vi "Read Tree Menu Plugin Entries.vi"(4 "Error In":errorcluster, 6 "Menu Context":T1, 7 "Config Data_DB_JET in":refnum<class "Config Data_DB_ADO_Jet.lvclass">) -> (0 "Error Out":errorcluster, 2 "Tree Menu Plugin Entries":T2[](array[typedef]), 3 "Config Data_DB_JET out":refnum<class "Config Data_DB_ADO_Jet.lvclass">)   [LabVIEW 2020, in "Config Data.lvlib" / "Config Data_DB_ADO_Jet.lvclass"]
uses:
  Config Data_DB_ADO_Jet.lvclass
  C:/Users/Fred Guo/Desktop/Release 19/_libraries/Config Data/DB/Config Data_DB.lvclass
  typedefs/Tree Menu Entry.ctl
  typedefs/Menu Context Selections.ctl
  toolbox/ADO Database Drivers/ADO Database Drivers.lvlib
  Config Data_DB.lvclass
  Config Data.lvclass
  Config Data_DB_ADO.lvclass
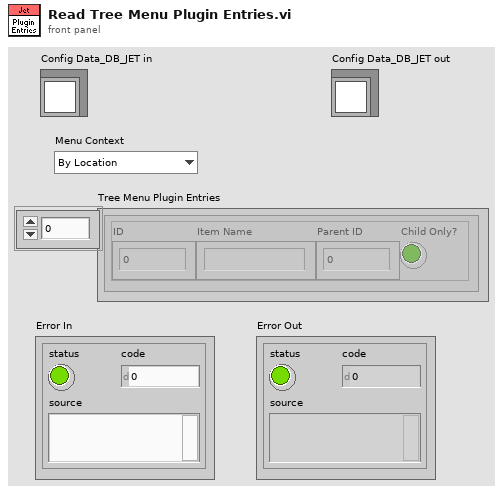
[diagram p1: front panel]
types:
  T1 = typedef "Config Data.lvlib/Config Data.lvclass/Menu Context Selections.ctl" = enum16{"By Location", "By Function"}
  T2 = typedef "Config Data.lvlib/Config Data.lvclass/Tree Menu Entry.ctl" = cluster{"ID":i32, "Item Name":string, "Parent ID":i32, "Child Only?":bool}
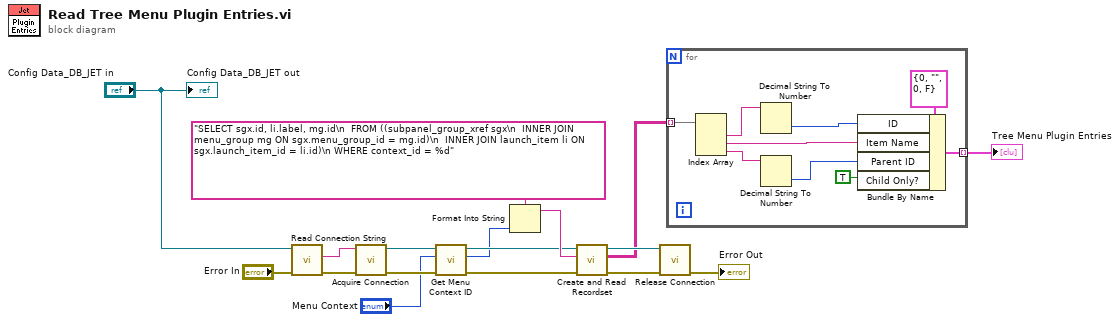
[diagram p0: block diagram]
diagram:
  n1 = call "Read Connection String.vi"("Error In"="Error In", "DB In"="Config Data_DB_JET in") -> ("Error Out"=w14:errorcluster, "Connection String"=w13:string)  [unwired: 3 in, 1 out]
  n2 = call "Acquire Connection.vi"("error in (no error)"=w14, "Connection String"=w13) -> ("error out"=w5:errorcluster, "Connection"=w6:refnum<k7>)  [unwired: 3 in, 1 out]
  n3 = call "Get Menu Context ID.vi"("error in (no error)"=w5, "Menu Context"="Menu Context", "Connection In"=w6) -> ("error out"=w4:errorcluster, "context_id"=w2:i32, "Connection Out"=w3:refnum<k7>)  [unwired: 2 in]
  n4 = Format Into String(format string="SELECT sgx.id, li.label, mg.id\n  FROM ((subpanel_group_xref sgx\n  INNER JOIN menu_group mg ON sgx.menu_group_id = mg.id)\n  INNER JOIN launch_item li ON sgx.launch_item_id = li.id)\n WHERE context_id = %d", w2) -> (resulting string=w12:string)  [unwired: 2 in, 1 out]
  n5 = call "Create and Read Recordset.vi"("error in (no error)"=w4, "Source"=w12, "Connection In"=w3) -> ("error out"=w17:errorcluster, "DB Data"=w10:string[][], "Connection Out"=w16:refnum<k7>)  [unwired: 2 in, 2 out]
  n6 = call "Release Connection.vi"("error in"=w17, "Connection"=w16) -> ("error out"=→"Error Out":errorcluster)  [unwired: 5 in]
  n7 = for {
    tunnel: w10 -> [w22] mode=indexing
    tunnel: [w18] -> w11 mode=indexing
    n8 = Index Array(array=w22) -> (element #1=w19:string, element #2=w21:string, element #3=w20:string)  [unwired: 3 in]
    n9 = Decimal String To Number(string=w19) -> (number=w25:i32)  [unwired: 2 in, 1 out]
    n10 = Decimal String To Number(string=w20) -> (number=w23:i32)  [unwired: 2 in, 1 out]
    n11 = Bundle By Name(cluster=T2 {"ID"=0, "Item Name"="", "Parent ID"=0, "Child Only?"=FALSE}, "ID"=w25, "Item Name"=w21, "Parent ID"=w23, "Child Only?"=TRUE) -> (w18:T2)
  }
  "Tree Menu Plugin Entries" <- w11
  "Config Data_DB_JET out" <- "Config Data_DB_JET in"
